vi "Time.Date Adjust.vi"(11 "Action":T1) -> (2 "End":timestamp, 3 "Start":timestamp)   [LabVIEW 2019]
uses:
  Time.Date Adjust Action.ctl
  Time.DateTime Adjust Action.ctl
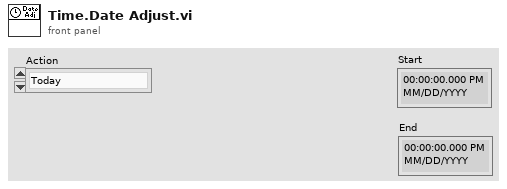
[diagram p1: front panel]
types:
  T1 = typedef "Time.Date Adjust Action.ctl" = enum16{"Today", "Yesterday", "This Week", "Last Week", "Last 2 Weeks", "Last 3 Weeks", "Last 4 Weeks"}
  T2 = typedef "Time.DateTime Adjust Action.ctl" = enum16{"Day Start", "Day End", "Offset Hrs", "UTC to Local", "Local to UTC"}
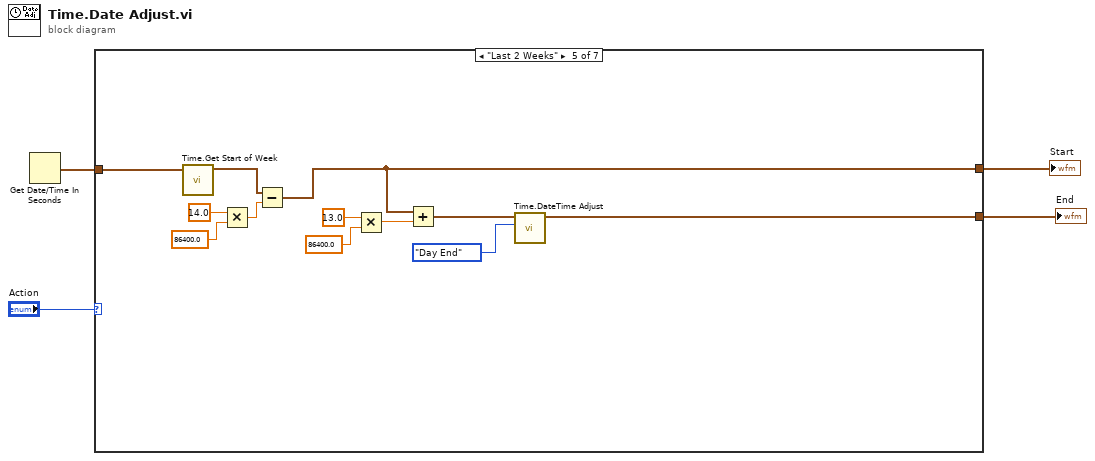
[diagram p0: block diagram]
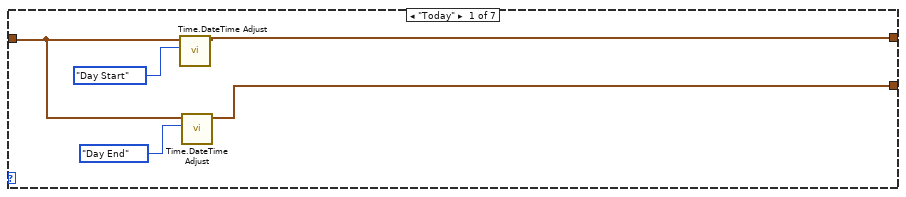
[diagram p2: hidden frame]
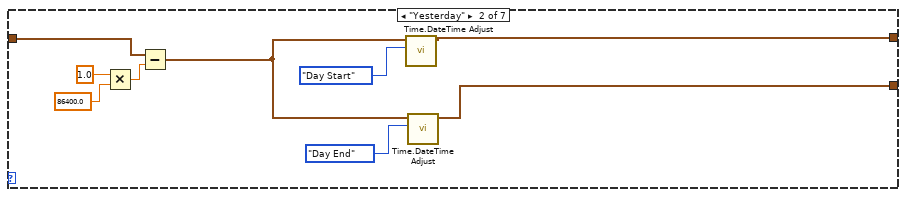
[diagram p3: hidden frame]
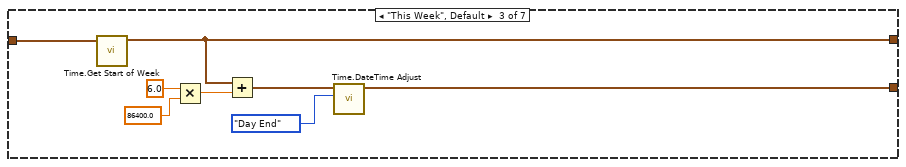
[diagram p4: hidden frame]
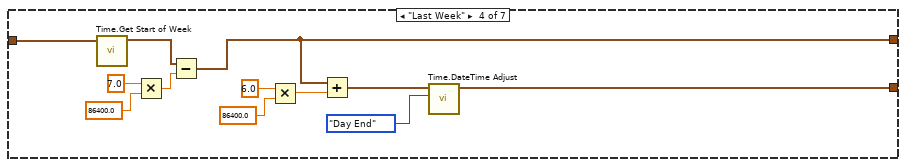
[diagram p5: hidden frame]
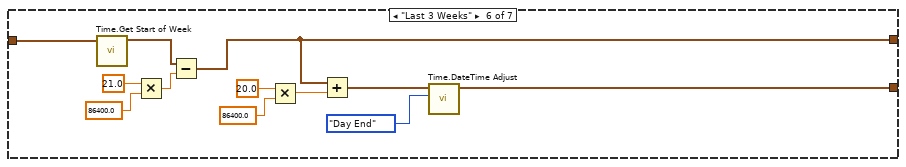
[diagram p6: hidden frame]
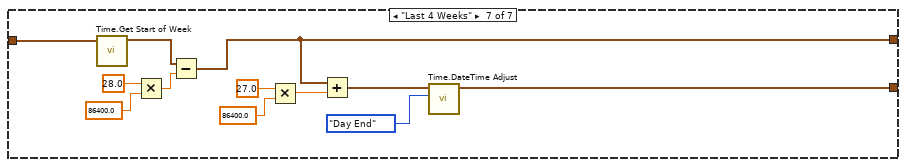
[diagram p7: hidden frame]
diagram:
  n1 = Get Date/Time In Seconds() -> (seconds since 1Jan1904=w2:timestamp)
  n2 = case shown="\"Last 2 Weeks\"" "Action" {
    tunnel: w2 -> [w7 w11 w25 w37 w49 w61 w73]
    tunnel: [w6 w16 w22 w27 w39 w51 w63] -> w3
    tunnel: [w5 w15 w19 w32 w44 w56 w68] -> w1
    frame "Today" {
      n3 = call "Time.DateTime Adjust.vi"("Action"=Time.DateTime_Adjust_Action."Day Start", "Time Stamp"=w7) -> ("Time Stamp Out"=w6:timestamp)  [unwired: 8 in, 1 out]
      n4 = call "Time.DateTime Adjust.vi"("Action"=Time.DateTime_Adjust_Action."Day End", "Time Stamp"=w7) -> ("Time Stamp Out"=w5:timestamp)  [unwired: 8 in, 1 out]
    }
    frame "Yesterday" {
      n5 = Multiply(x=1.0, y=86400.0) -> (x*y=w12:dbl)
      n6 = Subtract(x=w11, y=w12) -> (x-y=w10:timestamp)
      n7 = call "Time.DateTime Adjust.vi"("Action"=Time.DateTime_Adjust_Action."Day Start", "Time Stamp"=w10) -> ("Time Stamp Out"=w16:timestamp)  [unwired: 8 in, 1 out]
      n8 = call "Time.DateTime Adjust.vi"("Action"=Time.DateTime_Adjust_Action."Day End", "Time Stamp"=w10) -> ("Time Stamp Out"=w15:timestamp)  [unwired: 8 in, 1 out]
    }
    frame "This Week", Default {
      n9 = call "Time.Get Start of Week.vi"("Time In"=w25) -> ("Start of Week"=w22:timestamp)  [unwired: 10 in]
      n10 = Multiply(x=6.0, y=86400.0) -> (x*y=w23:dbl)
      n11 = Add(x=w22, y=w23) -> (x+y=w21:timestamp)
      n12 = call "Time.DateTime Adjust.vi"("Action"=Time.DateTime_Adjust_Action."Day End", "Time Stamp"=w21) -> ("Time Stamp Out"=w19:timestamp)  [unwired: 8 in, 1 out]
    }
    frame "Last Week" {
      n13 = call "Time.Get Start of Week.vi"("Time In"=w37) -> ("Start of Week"=w29:timestamp)  [unwired: 10 in]
      n14 = Multiply(x=7.0, y=86400.0) -> (x*y=w28:dbl)
      n15 = Subtract(x=w29, y=w28) -> (x-y=w27:timestamp)
      n16 = Multiply(x=6.0, y=86400.0) -> (x*y=w35:dbl)
      n17 = Add(x=w27, y=w35) -> (x+y=w34:timestamp)
      n18 = call "Time.DateTime Adjust.vi"("Action"=Time.DateTime_Adjust_Action."Day End", "Time Stamp"=w34) -> ("Time Stamp Out"=w32:timestamp)  [unwired: 8 in, 1 out]
    }
    frame "Last 2 Weeks" {
      n19 = call "Time.Get Start of Week.vi"("Time In"=w49) -> ("Start of Week"=w41:timestamp)  [unwired: 10 in]
      n20 = Multiply(x=14.0, y=86400.0) -> (x*y=w40:dbl)
      n21 = Subtract(x=w41, y=w40) -> (x-y=w39:timestamp)
      n22 = Multiply(x=13.0, y=86400.0) -> (x*y=w47:dbl)
      n23 = Add(x=w39, y=w47) -> (x+y=w46:timestamp)
      n24 = call "Time.DateTime Adjust.vi"("Action"=Time.DateTime_Adjust_Action."Day End", "Time Stamp"=w46) -> ("Time Stamp Out"=w44:timestamp)  [unwired: 8 in, 1 out]
    }
    frame "Last 3 Weeks" {
      n25 = call "Time.Get Start of Week.vi"("Time In"=w61) -> ("Start of Week"=w53:timestamp)  [unwired: 10 in]
      n26 = Multiply(x=21.0, y=86400.0) -> (x*y=w52:dbl)
      n27 = Subtract(x=w53, y=w52) -> (x-y=w51:timestamp)
      n28 = Multiply(x=20.0, y=86400.0) -> (x*y=w59:dbl)
      n29 = Add(x=w51, y=w59) -> (x+y=w58:timestamp)
      n30 = call "Time.DateTime Adjust.vi"("Action"=Time.DateTime_Adjust_Action."Day End", "Time Stamp"=w58) -> ("Time Stamp Out"=w56:timestamp)  [unwired: 8 in, 1 out]
    }
    frame "Last 4 Weeks" {
      n31 = call "Time.Get Start of Week.vi"("Time In"=w73) -> ("Start of Week"=w65:timestamp)  [unwired: 10 in]
      n32 = Multiply(x=28.0, y=86400.0) -> (x*y=w64:dbl)
      n33 = Subtract(x=w65, y=w64) -> (x-y=w63:timestamp)
      n34 = Multiply(x=27.0, y=86400.0) -> (x*y=w71:dbl)
      n35 = Add(x=w63, y=w71) -> (x+y=w70:timestamp)
      n36 = call "Time.DateTime Adjust.vi"("Action"=Time.DateTime_Adjust_Action."Day End", "Time Stamp"=w70) -> ("Time Stamp Out"=w68:timestamp)  [unwired: 8 in, 1 out]
    }
  }
  "Start" <- w3
  "End" <- w1
